vi "Global 1.vi"() -> ()   [LabVIEW 2019]
panel:
  in  "Boolean":bool
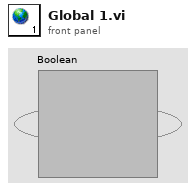
[diagram p1: front panel]
diagram:
